vi "Timestamp to Unix Time.vi"(11 "Timestamp (now)":timestamp) -> (2 "Fractional Second":dbl, 3 "Unix Time (s)":i64)   [LabVIEW 2021]
uses:
  Epoch.UNIX.lvclass
  C:/Users/Fujitsu/Desktop/Nouveau dossier/avril/Project mqtt/Epoch Date & Time/epoch/Epoch.lvclass
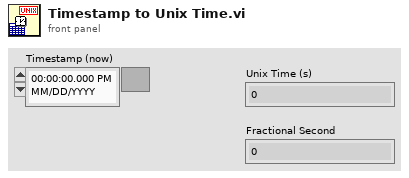
[diagram p1: front panel]
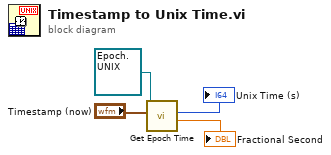
[diagram p0: block diagram]
diagram:
  n1 = call "Get Epoch Time.vi"("Timestamp (now)"="Timestamp (now)", "Epoch (Local)"=refnum<class "Epoch.UNIX.lvclass"> refnum ("Epoch.UNIX.lvclass")) -> ("Fractional Second"=→"Fractional Second":dbl, "Epoch Time (s)"=→"Unix Time (s)":i64)  [unwired: 7 in, 1 out]
